vi "DSF.Engine.Transfer.Set DBL Buffer.vi"(10 "DBL Buffer":refnum<class "DSF.Engine.Pointer.DBL.lvclass">, 11 "Transfer in":refnum<class "DSF.Engine.Transfer.lvclass">) -> (3 "Transfer out":refnum<class "DSF.Engine.Transfer.lvclass">)   [LabVIEW 2017, in "DSF.Engine.lvlib" / "DSF.Engine.Transfer.lvclass"]
uses:
  DSF.Engine.Transfer.lvclass
  Pointer/DSF.Engine.Pointer.DBL.lvclass
  DSF.Engine.Transfer.lvclass/DSF.Engine.Transfer.ctl
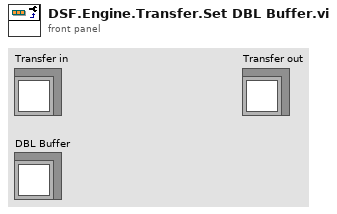
[diagram p1: front panel]
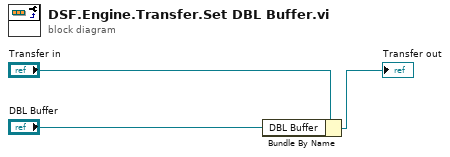
[diagram p0: block diagram]
diagram:
  n1 = Bundle By Name(cluster="Transfer in", "DBL Buffer"="DBL Buffer") -> (→"Transfer out":refnum<class "DSF.Engine.Transfer.lvclass">)
